vi "PicoScope4000WrapSettings.vi"(7 "Unit Info":T1, 8 "error in (no error)":errorcluster, 9 "Enabled array":i16[](array[numeric]), 11 "Handle In":i16) -> (0 "error out":errorcluster, 3 "Handle Out":i16)   [LabVIEW 2009]
uses:
  ps4000Wrap.dll
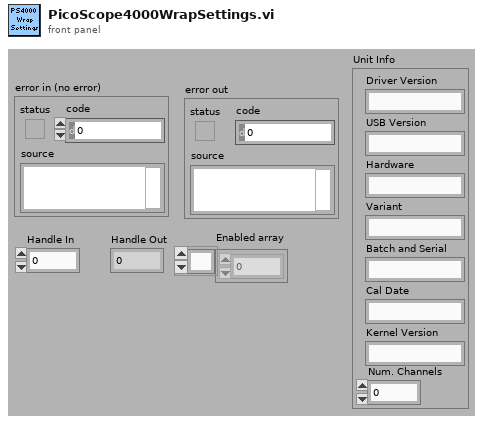
[diagram p1: front panel]
types:
  T1 = cluster{"Driver Version":string, "USB Version":string, "Hardware":string, "Variant":string, "Batch and Serial":string, "Cal Date":string, "Kernel Version":string, "Num. Channels":i16}
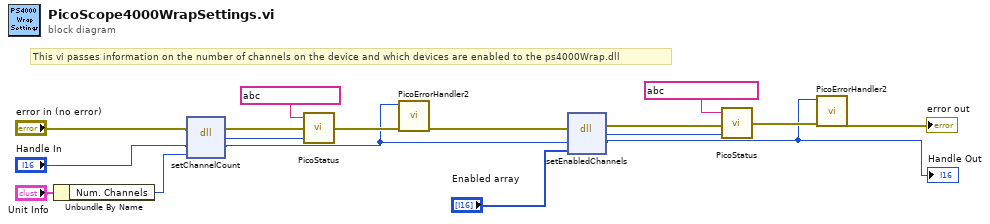
[diagram p0: block diagram]
diagram:
  # "This vi passes information on the number of channels on the device and which devices are enabled to the ps4000Wrap.dll"
  n1 = Unbundle By Name("Unit Info") -> ("Num. Channels"=w13:i16)
  n2 = dll-call lib="ps4000Wrap.dll" fn="setChannelCount"(error in="error in (no error)", "handle"="Handle In", "channelCount"=w13) -> (error out=w8:errorcluster, "PICO_STATUS"=w7:u32, "handle"=w3:i16)  [unwired: 3 in, 1 out]
  n3 = call "PicoStatus.vi"("PICO STATUS"=w7, "error in"=w8, "source"=string ?) -> ("error out"=w12:errorcluster)
  n4 = call "PicoErrorHandler2.vi"("error in (no error)"=w12, "handle In"=w3) -> ("error out"=w6:errorcluster)  [unwired: 9 in]
  n5 = dll-call lib="ps4000Wrap.dll" fn="setEnabledChannels"(error in=w6, "handle"=w3, "enabledChannels"="Enabled array") -> (error out=w5:errorcluster, "PICO_STATUS"=w4:u32, "handle"=w2:i16)  [unwired: 3 in, 1 out]
  "Handle Out" <- w2
  n6 = call "PicoStatus.vi"("PICO STATUS"=w4, "error in"=w5, "source"=string ?) -> ("error out"=w11:errorcluster)
  n7 = call "PicoErrorHandler2.vi"("error in (no error)"=w11, "handle In"=w2) -> ("error out"=→"error out":errorcluster)  [unwired: 9 in]
